vi "Connect.vi"(8 "Error In":errorcluster, 11 "Agent In":refnum<class "Agent.lvclass">) -> (0 "Error Out":errorcluster, 3 "Agent Out":refnum<class "Agent.lvclass">)   [LabVIEW 2021, in "Field_RnD_Services_LIBSSH2_Toolkit.lvlib" / "Agent.lvclass"]
doc: "Establish a connection with a running SSH-agent application. This must be called before requesting the list of identities that are available for logging into a remote SSH server with the First Identity VI."
uses:
  220524-VNA RP FLAT.llb/Agent.lvclass
  220524-VNA RP FLAT.llb/Agent.lvclass/Agent.ctl
  220524-VNA RP FLAT.llb/Field_RnD_Services_LIBSSH2_Toolkit.lvlib
  220524-VNA RP FLAT.llb/Session.lvclass
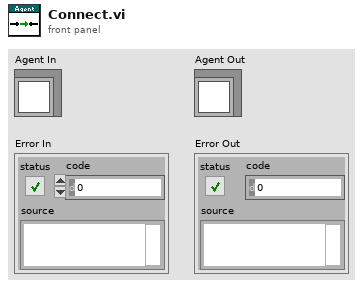
[diagram p1: front panel]
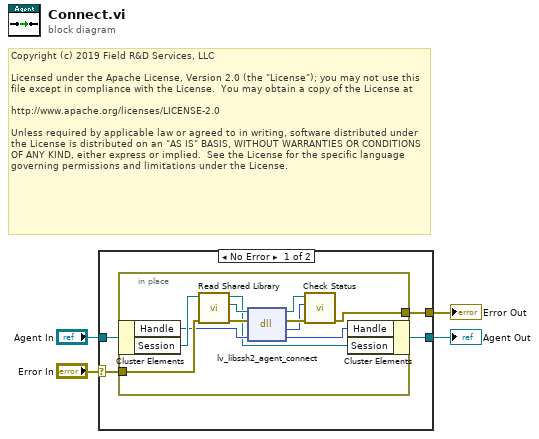
[diagram p0: block diagram]
diagram:
  # "Copyright (c) 2019 Field R&D Services, LLC\n\nLicensed under the Apache License, Version 2.0 (the \"License\"); you may not use this file except in compliance with the License.  You may obtain a copy of the License at\n\nhttp://www.apache.org/licenses/LICENSE-2.0\n\nUnless required by applicable law or agreed to in writing, software distributed under the License is distributed on an \"AS IS\" BASIS, WITHOUT WARRANTIES OR CONDITIONS OF ANY KIND, either express or implied.  See the License for the specific language governing permissions and limitations under the License."
  n1 = case shown="No Error" "Error In" {
    selector: "Error In" -> [w7 w21]
    tunnel: [w8 w21] -> w3
    tunnel: "Agent In" -> [w6 w20]
    tunnel: [w5 w20] -> w1
    frame No Error {
      n2 = in-place {
        in-place-border: [w16] -> w8
        in-place-border: w7 -> [w11]
        n3 = in-place-cluster #1(w6) -> ("Handle"=w10:u64, "Session"=w14:refnum<class "Session.lvclass">)
        n4 = call "Read Shared Library.vi"("Error In"=w11, "Session In"=w14) -> ("Erorr Out"=w12:errorcluster, "libssh2lv Shared Library"=w13:path, "Session Out"=w9:refnum<class "Session.lvclass">)  [unwired: 7 in]
        n5 = dll-call lib="libssh2lv.*" fn="lv_libssh2_agent_connect"(path in=w13, error in=w12, "handle"=w10) -> (path out=w17:path, error out=w18:errorcluster, "result"=w15:i32, "handle"=w19:u64)  [unwired: 1 in]
        n6 = call "Check Status.vi"("Error In"=w18, "Status"=w15, "libssh2lv Shared Library In"=w17) -> ("Error Out"=w16:errorcluster)  [unwired: 7 in, 1 out]
        n7 = in-place-cluster #1("Handle"=w19, "Session"=w9) -> (w5:refnum<class "Agent.lvclass">)
      }
    }
    frame Error {
    }
  }
  "Error Out" <- w3
  "Agent Out" <- w1
